vi "DexPropertyNode.vi"   [LabVIEW 2017]
doc: "Gets (reads) and/or sets (writes) properties of a reference."
uses:
  <resource>/objmgr/ni.dex.rc
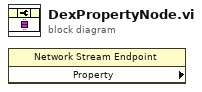
[diagram p0: block diagram]
diagram:
  n1 = property class="Network Stream Endpoint" props=[]() -> ()  [unwired: 2 in, 3 out]
